vi "UPFAIL.vi"(0 "总成追溯码":string, 1 "产品型号":string, 5 "不合格代码":string, 7 "操作员":string, 9 "下线位置":string, 11 "错误输入":errorcluster, 12 "工位追溯码":string) -> (15 "错误输出":errorcluster)   [LabVIEW 2018]
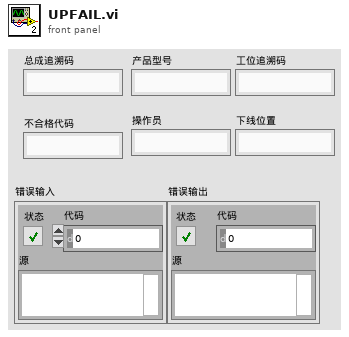
[diagram p1: front panel]
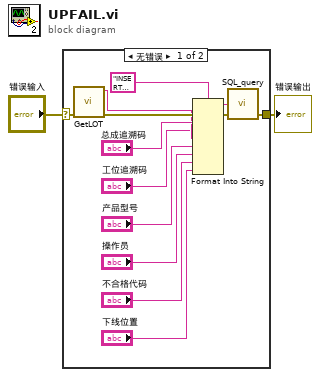
[diagram p0: block diagram]
diagram:
  n1 = case shown="无错误" "错误输入" {
    selector: "错误输入" -> [w11 w16]
    tunnel: [w12 w16] -> w1
    frame No Error {
      n2 = call "GetLOT.vi"("错误输入"=w11) -> ("错误输出"=w10:errorcluster, "LOT"=w5:string)  [unwired: 8 in, 1 out]
      n3 = Format Into String(format string="INSERT INTO [SanliServer].[dbo].[不合格] (\n\t[总成追溯码],\n [工位追溯码],\n\t[生产编号],\n\t[产品型号],\n\t[操作员],\n\t[不合格代码],\n\t[下线位置]\n)VALUES\n\t(\n\t\tN'%s',\n\t\tN'%s',\n\t\tN'%s',\n\t\tN'%s',\n\t\tN'%s',\n\t\tN'%s',\n\t\tN'%s'\n\t)", error in=w10, "总成追溯码", "工位追溯码", w5, "产品型号", "操作员", "不合格代码", "下线位置") -> (resulting string=w14:string, error out=w13:errorcluster)  [unwired: 1 in]
      n4 = call "SQL_query.vi"("error in (no error)"=w13, "SQL query"=w14) -> ("error out"=w12:errorcluster)  [unwired: 1 in, 2 out]
    }
    frame Error {
    }
  }
  "错误输出" <- w1
